vi "Remove Pending Transfer.vi"(8 "error in":errorcluster, 10 "SDO Transfer":refnum<class "SDO Transfer.lvclass">, 11 "Pending Transfers":refnum<data-value>) -> (0 "error out":errorcluster, 2 "Removed SDO Transfer":refnum<class "SDO Transfer.lvclass">)   [LabVIEW 2020, in "CANopen.lvlib" / "SDO Manager.lvlib" / "SDO Manager.lvclass"]
uses:
  SDO Manager.lvclass
  SDO Transfer/SDO Transfer.lvclass
  SDO Transfer/SDO Transfer.lvclass/SDO Transfer.ctl
  SDO Manager.lvclass/SDO Manager.ctl
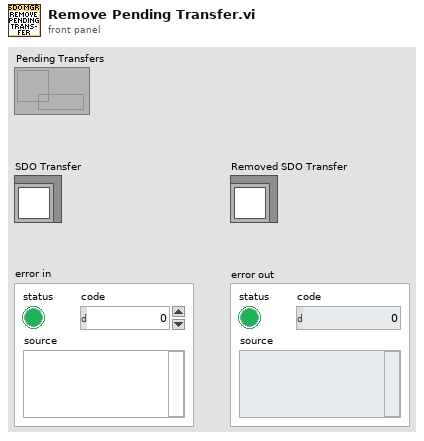
[diagram p1: front panel]
types:
  T1 = map{string, refnum<class "SDO Transfer.lvclass">}
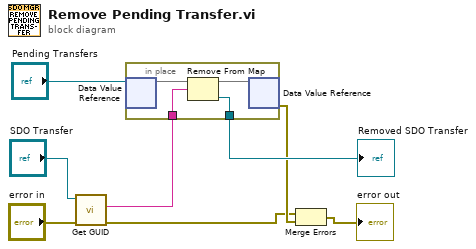
[diagram p0: block diagram]
diagram:
  n1 = call "Get GUID.vi"("error in"="error in", "SDO Transfer in"="SDO Transfer") -> ("error out"=w3:errorcluster, "GUID"=w1:string)  [unwired: 7 in, 1 out]
  n2 = in-place {
    in-place-border: [w10] -> w8
    in-place-border: w1 -> [w9]
    n3 = in-place-dvr #1("Pending Transfers") -> (w12:T1)  [unwired: 1 out]
    n4 = Remove From Map(10:w9, 11:w12) -> (1:w10:refnum<class "SDO Transfer.lvclass">, 3:w11:T1)  [unwired: 1 out]
    n5 = in-place-dvr #1(w11) -> (w4:errorcluster)  [unwired: 1 out]
  }
  "Removed SDO Transfer" <- w8
  n6 = Merge Errors(w3, w4) -> (→"error out":errorcluster)
